vi "GermanInfo_settings_ut_test.vi"(8 "Error In":errorcluster, 11 "Germaninfo in":T1 {"Окно с настройками"."scheme" items=["Complete test scheme 1", "Complete test scheme 2", "Complete test scheme 3"]}) -> (0 "Error Out":errorcluster, 3 "Germaninfo out":T1 {"Окно с настройками"."scheme" items=["Complete test scheme 1", "Complete test scheme 2", "Complete test scheme 3"]})   [LabVIEW 2018]
uses:
  GermanInfo.ctl
  MOKO_LabViewLibrary/MokoSTM/MokoClassicUtilitySTM/MCUS_STM.ctl
  MOKO_LabViewLibrary/MokoSTM/MokoClassicUtilitySTM/MCUS_ITEM.ctl
  <vilib>/addons/_JKI.lib/Serialization/JSON/JKI JSON Serialization.lvlib
panel:
  in  "Iout_EL":dbl=1.0
  in  "Uout_EL":dbl=1.0
  in  "Iin_PS":dbl=1.0
  in  "Reset":bool
  in  "Open":bool
  in  "Save":bool
  in  "Setting Path":path
  in  "Применить":bool
  in  "Uin_PS":dbl=1.0
  in  "Scheme":u16(ring) items=["Complete test scheme 1", "Complete test scheme 2", "Complete test scheme 3"]
  # "Входное напряжение (Uin_PS):"
  # "Входной ток (Iin_PS):"
  # "0,4\n0,6\n1\n1,5\n1,6\n2,5\n4"
  # "kPa\nbar\nkgf/cm2\nMPa"
  # "Выходное напряжение (Uout_EL):"
  # "Выходной ток (Iout_EL):"
  # "Схема измерений:"
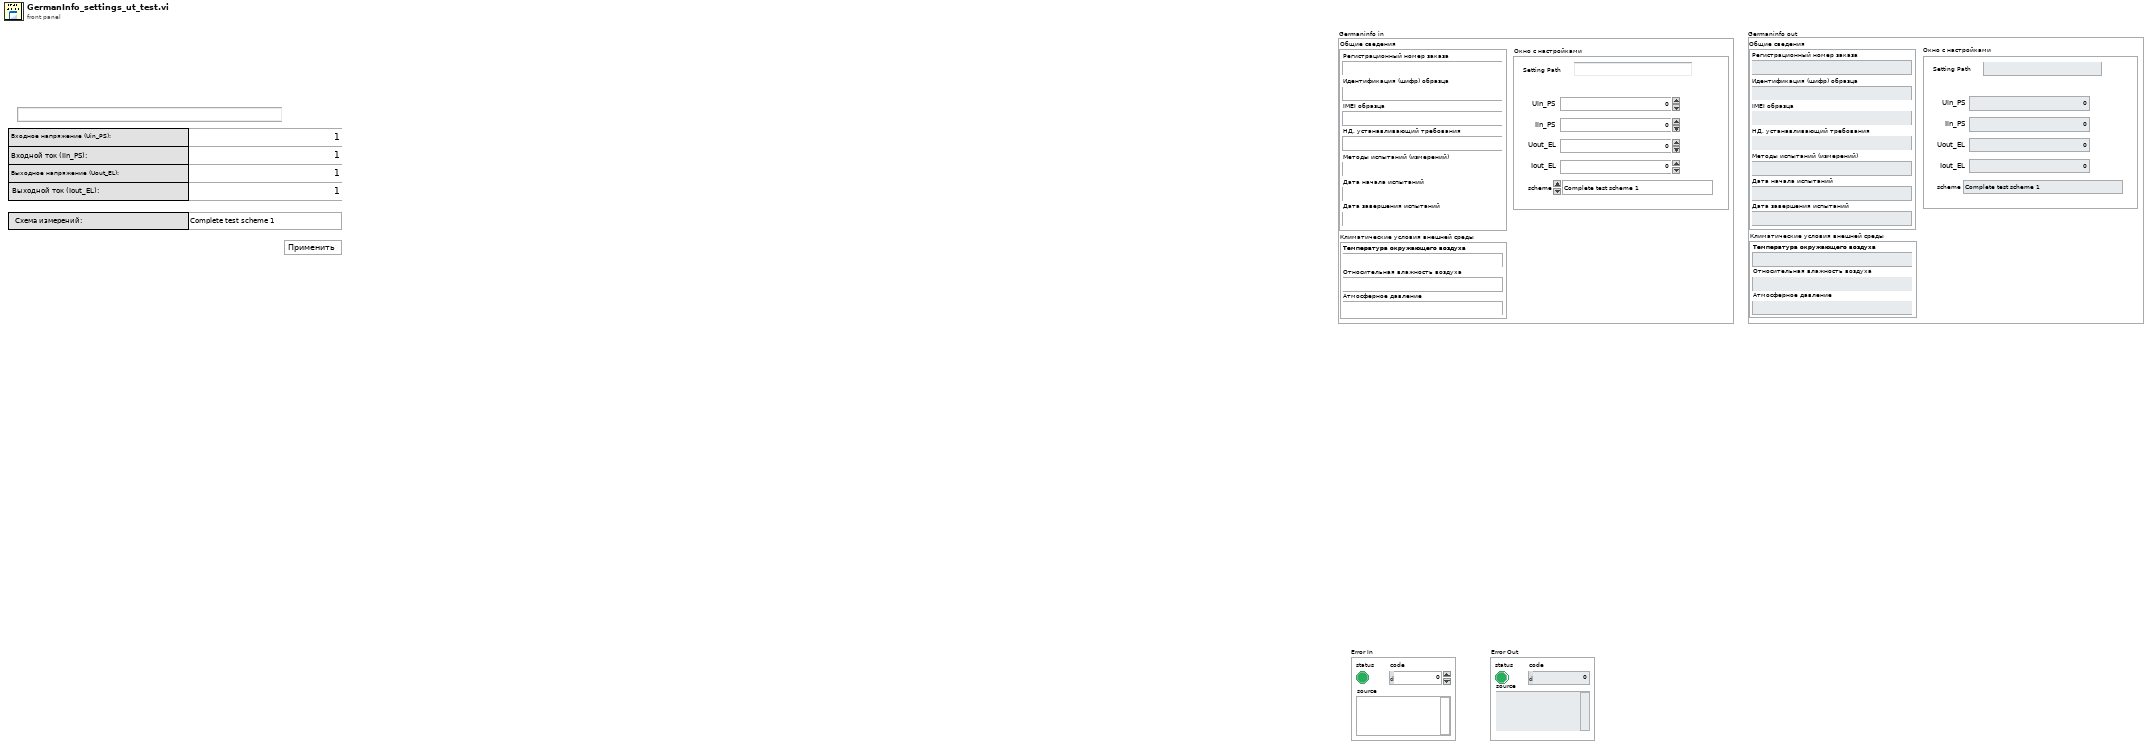
[diagram p1: front panel]
types:
  T1 = typedef "GermanInfo.ctl" = cluster{"Общие сведения":cluster{"Регистрационный номер заказа":string, "Идентификация (шифр) образца":string, "IMEI образца":string, "НД, устанавливающий требования":string, "Методы испытаний (измерений)":string, "Дата начала испытаний":string, "Дата завершения испытаний":string}, "Климатические условия внешней среды":cluster{"Температура окружающего воздуха":string, "Относительная влажность воздуха":string, "Атмосферное давление":string}, "Окно с настройками":cluster{"Uin_PS":dbl, "Setting Path":path, "Iin_PS":dbl, "Uout_EL":dbl, "Iout_EL":dbl, "scheme":u16}}
  T2 = typedef "MCUS_STM.ctl" = cluster{"main stm":T3, "data":string}
  T3 = typedef "MCUS_ITEM.ctl" = enum16{"idle", "_____ main_____ ", "Init", "Stop", "Apply values", "Save", "Open", "Reset"}
  T4 = cluster{"Uin_PS":dbl, "Setting Path":path, "Iin_PS":dbl, "Uout_EL":dbl, "Iout_EL":dbl, "scheme":u16}
  T5 = enum16{"open", "replace", "create", "open or create", "replace or create", "replace or create with confirmation"}
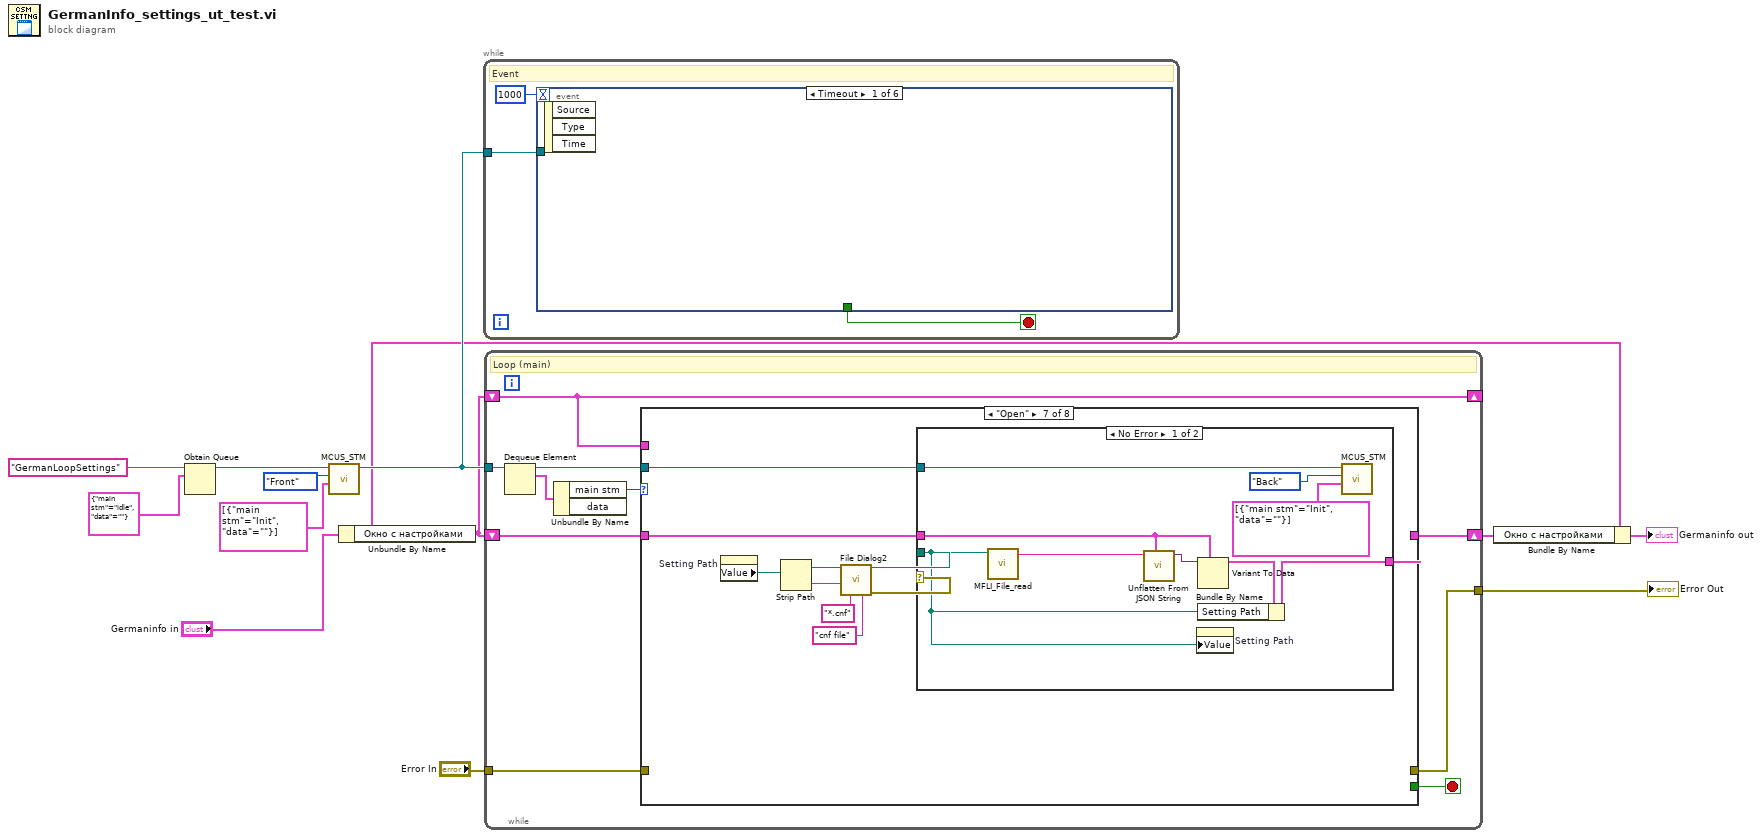
[diagram p0: block diagram]
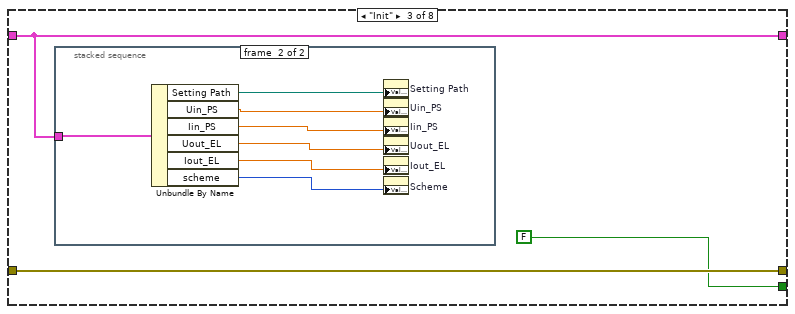
[diagram p4: hidden frame]
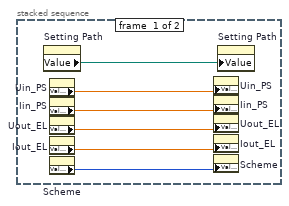
[diagram p5: hidden frame]
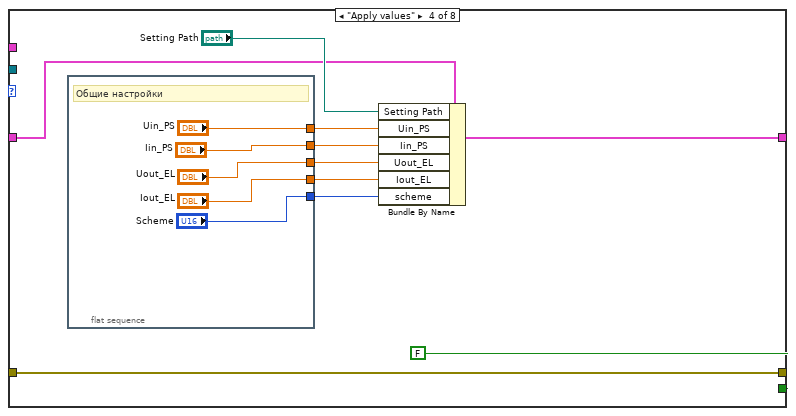
[diagram p6: hidden frame]
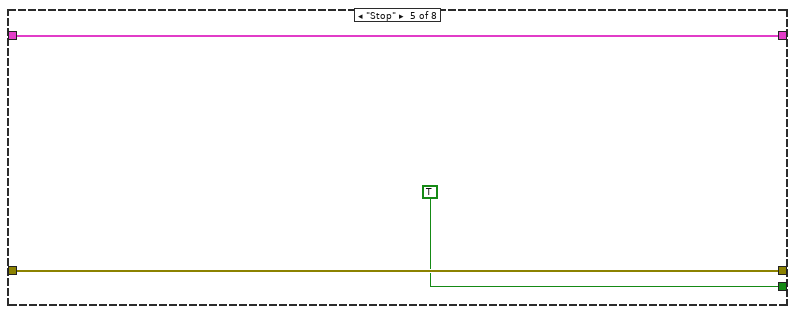
[diagram p7: hidden frame]
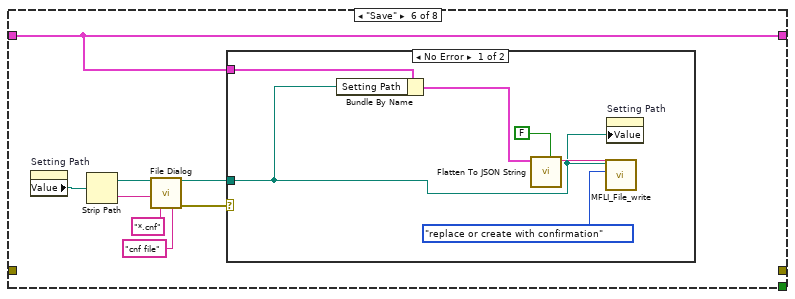
[diagram p8: hidden frame]
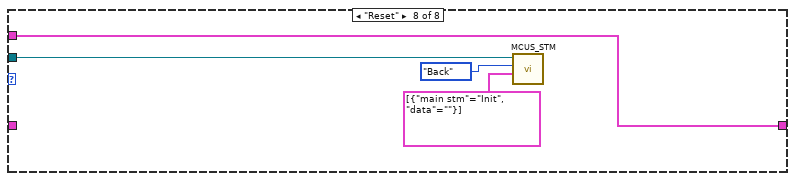
[diagram p11: hidden frame]
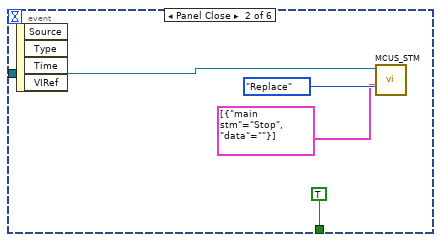
[diagram p12: hidden frame]
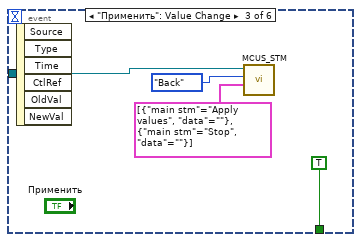
[diagram p13: hidden frame]
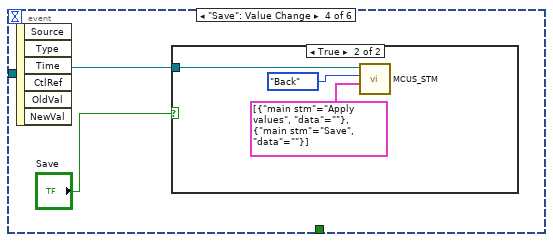
[diagram p14: hidden frame]
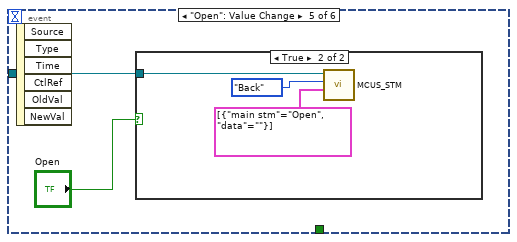
[diagram p16: hidden frame]
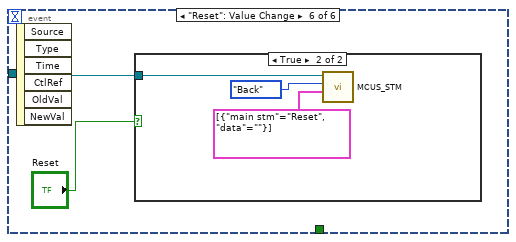
[diagram p18: hidden frame]
diagram:
  n1 = Obtain Queue(name (unnamed)="GermanLoopSettings", element data type=T2 {"main stm"=enum."idle", "data"=""} ("MOKO_NMEA")) -> (queue out=w12:refnum<queue>)  [unwired: 3 in, 2 out]
  n2 = call "MCUS_STM.vi"("StateMachineSteps"=T2[] [{"main stm"=enum."Init", "data"=""}], "FNs"=enum16{"Back", "Front", "Replace"}."Front", "Queue in"=w12) -> ("Queue out"=w7:refnum<queue>)  [unwired: 7 in, 1 out]
  n3 = Unbundle By Name("Germaninfo in") -> ("Окно с настройками"=w4:T4)
  n4 = while {
    tunnel: w7 -> [w13]
    stop <- w15 stop-if-true
    # "Event"
    n5 = event shown="[0] Timeout" {
      selector: _ -> [_ _ _ _ _ _]
      dyn-events: _ -> [_ _ _ _ _ _]
      timeout: 1000 -> [_ _ _ _ _ _]
      tunnel: [_ TRUE TRUE _ _ _] -> w15
      tunnel: w13 -> [_ w16 w21 w25 w30 w35]
      event Timeout {
        n6 = event-data() -> ()  [unwired: 1 in, 3 out]
      }
      event Panel Close {
        n7 = event-data() -> ()  [unwired: 1 in, 4 out]
        n8 = call "MCUS_STM.vi"("StateMachineSteps"=T2[] [{"main stm"=enum."Stop", "data"=""}], "FNs"=enum16{"Back", "Front", "Replace"}."Replace", "Queue in"=w16) -> ()  [unwired: 7 in, 2 out]
      }
      event "Применить": Value Change {
        n9 = event-data() -> ()  [unwired: 1 in, 6 out]
        n10 = call "MCUS_STM.vi"("StateMachineSteps"=T2[] [{"main stm"=enum."Apply values", "data"=""}, {"main stm"=enum."Stop", "data"=""}], "FNs"=enum16{"Back", "Front", "Replace"}."Back", "Queue in"=w21) -> ()  [unwired: 7 in, 2 out]
      }
      event "Save": Value Change {
        n11 = event-data() -> ()  [unwired: 1 in, 6 out]
        n12 = case shown="True" "Save" {
          tunnel: w25 -> [_ w26]
          frame False {
          }
          frame True {
            n13 = call "MCUS_STM.vi"("StateMachineSteps"=T2[] [{"main stm"=enum."Apply values", "data"=""}, {"main stm"=enum."Save", "data"=""}], "FNs"=enum16{"Back", "Front", "Replace"}."Back", "Queue in"=w26) -> ()  [unwired: 7 in, 2 out]
          }
        }
      }
      event "Open": Value Change {
        n14 = event-data() -> ()  [unwired: 1 in, 6 out]
        n15 = case shown="True" "Open" {
          tunnel: w30 -> [_ w31]
          frame False {
          }
          frame True {
            n16 = call "MCUS_STM.vi"("StateMachineSteps"=T2[] [{"main stm"=enum."Open", "data"=""}], "FNs"=enum16{"Back", "Front", "Replace"}."Back", "Queue in"=w31) -> ()  [unwired: 7 in, 2 out]
          }
        }
      }
      event "Reset": Value Change {
        n17 = event-data() -> ()  [unwired: 1 in, 6 out]
        n18 = case shown="True" "Reset" {
          tunnel: w35 -> [_ w36]
          frame False {
          }
          frame True {
            n19 = call "MCUS_STM.vi"("StateMachineSteps"=T2[] [{"main stm"=enum."Reset", "data"=""}], "FNs"=enum16{"Back", "Front", "Replace"}."Back", "Queue in"=w36) -> ()  [unwired: 7 in, 2 out]
          }
        }
      }
    }
  }
  n20 = while {
    tunnel: w7 -> [w48]
    tunnel: "Error In" -> [w44]
    tunnel: [w43] -> w5
    shift-right: [w42] -> w2
    shift-left: w4 -> [w40]
    shift-right: [w39] -> _
    shift-left: w4 -> [w39]
    stop <- w45 stop-if-true
    # "Loop (main)"
    n21 = Dequeue Element(queue=w48) -> (queue out=w41:refnum<queue>, element=w47:T2)  [unwired: 2 in, 2 out]
    n22 = Unbundle By Name(w47) -> ("main stm"=w46:T3)  [unwired: 1 out]
    n23 = case shown="\"Open\"" w46 {
      tunnel: w41 -> [_ _ _ _ _ _ w104 w121]
      tunnel: [_ _ FALSE FALSE TRUE _ _ _] -> w45
      tunnel: w44 -> [w50 w52 w55 w78 w86 _ _ _]
      tunnel: [w50 w52 w55 w78 w86 _ _ _] -> w43
      tunnel: [w49 w51 w53 w76 w84 w90 w106 w124] -> w42
      tunnel: w40 -> [w49 w51 w53 w74 w84 w90 w105 _]
      tunnel: w39 -> [_ _ _ _ _ _ _ w124]
      frame "idle", Default {
      }
      frame "_____ main_____ " {
      }
      frame "Init" {
        n24 = stacked-sequence {
          tunnel: w53 -> [_ w68]
          frame #0 {
            n25 = property on="Setting Path" class="Path"() -> ("Value"=w61:path)  [unwired: 2 in, 2 out]
            n26 = property on="Uin_PS" class="DigNum (strict)"() -> ("Value"=w56:dbl)  [unwired: 2 in, 2 out]
            n27 = property on="Iin_PS" class="DigNum (strict)"() -> ("Value"=w57:dbl)  [unwired: 2 in, 2 out]
            n28 = property on="Uout_EL" class="DigNum (strict)"() -> ("Value"=w58:dbl)  [unwired: 2 in, 2 out]
            n29 = property on="Iout_EL" class="DigNum (strict)"() -> ("Value"=w59:dbl)  [unwired: 2 in, 2 out]
            n30 = property on="Scheme" class="Ring (strict)"() -> ("Value"=w60:u16)  [unwired: 2 in, 2 out]
            n31 = property on="Uin_PS" class="DigNum (strict)"("Value"=w56) -> ()  [unwired: 2 in, 2 out]
            n32 = property on="Iin_PS" class="DigNum (strict)"("Value"=w57) -> ()  [unwired: 2 in, 2 out]
            n33 = property on="Uout_EL" class="DigNum (strict)"("Value"=w58) -> ()  [unwired: 2 in, 2 out]
            n34 = property on="Iout_EL" class="DigNum (strict)"("Value"=w59) -> ()  [unwired: 2 in, 2 out]
            n35 = property on="Scheme" class="Ring (strict)"("Value"=w60) -> ()  [unwired: 2 in, 2 out]
            n36 = property on="Setting Path" class="Path"("Value"=w61) -> ()  [unwired: 2 in, 2 out]
          }
          frame #1 {
            n37 = Unbundle By Name(w68) -> ("Setting Path"=w67:path, "Uin_PS"=w65:dbl, "Iin_PS"=w64:dbl, "Uout_EL"=w63:dbl, "Iout_EL"=w62:dbl, "scheme"=w66:u16)
            n38 = property on="Setting Path" class="Path"("Value"=w67) -> ()  [unwired: 2 in, 2 out]
            n39 = property on="Uin_PS" class="DigNum (strict)"("Value"=w65) -> ()  [unwired: 2 in, 2 out]
            n40 = property on="Iin_PS" class="DigNum (strict)"("Value"=w64) -> ()  [unwired: 2 in, 2 out]
            n41 = property on="Uout_EL" class="DigNum (strict)"("Value"=w63) -> ()  [unwired: 2 in, 2 out]
            n42 = property on="Iout_EL" class="DigNum (strict)"("Value"=w62) -> ()  [unwired: 2 in, 2 out]
            n43 = property on="Scheme" class="Ring (strict)"("Value"=w66) -> ()  [unwired: 2 in, 2 out]
          }
        }
      }
      frame "Apply values" {
        n44 = flat-sequence {
          tunnel: ["Scheme"] -> w73
          tunnel: ["Uin_PS"] -> w72
          tunnel: ["Iin_PS"] -> w71
          tunnel: ["Uout_EL"] -> w70
          tunnel: ["Iout_EL"] -> w69
          frame #0 {
            # "Общие настройки"
          }
        }
        n45 = Bundle By Name(cluster=w74, "Setting Path"="Setting Path", "Uin_PS"=w72, "Iin_PS"=w71, "Uout_EL"=w70, "Iout_EL"=w69, "scheme"=w73) -> (w76:T4)
      }
      frame "Stop" {
      }
      frame "Save" {
        n46 = property on="Setting Path" class="Path"() -> ("Value"=w89:path)  [unwired: 2 in, 2 out]
        n47 = Strip Path(path=w89) -> (stripped path=w88:path, name=w87:string)
        n48 = call "File Dialog"("start path"=w88, "default name"=w87, "pattern (all files)"="*.cnf", "pattern label"="cnf file") -> ("selected path"=w92:path, "error out"=w91:errorcluster)  [unwired: 8 in, 2 out]
        n49 = case shown="No Error" w91 {
          tunnel: w90 -> [w97 _]
          tunnel: w92 -> [w96 _]
          frame No Error {
            n50 = Bundle By Name(cluster=w97, "Setting Path"=w96) -> (w95:T4)
            n51 = call <vilib>:"Flatten To JSON String.vi"("Numeric Extensions (F)"=FALSE, "Variant"=w95) -> ("JSON String"=w99:string)  [unwired: 8 in, 1 out]
            n52 = call "MFLI_File_write.vi"("String"=w99, "operation (0:open)"=T5."replace or create with confirmation", "selected path"=w96) -> ()  [unwired: 7 in, 2 out]
            n53 = property on="Setting Path" class="Path"("Value"=w96) -> ()  [unwired: 2 in, 2 out]
          }
          frame Error {
          }
        }
      }
      frame "Open" {
        n54 = property on="Setting Path" class="Path"() -> ("Value"=w103:path)  [unwired: 2 in, 2 out]
        n55 = Strip Path(path=w103) -> (stripped path=w101:path, name=w102:string)
        n56 = call "File Dialog2"("start path"=w101, "default name"=w102, "pattern (all files)"="*.cnf", "pattern label"="cnf file") -> ("selected path"=w108:path, "error out"=w107:errorcluster)  [unwired: 8 in, 2 out]
        n57 = case shown="No Error" w107 {
          tunnel: w108 -> [w111 _]
          tunnel: w104 -> [w117 _]
          tunnel: w105 -> [w115 w120]
          tunnel: [w112 w120] -> w106
          frame No Error {
            n58 = call "MFLI_File_read.vi"("Project script or program"=w111) -> ("String"=w116:string)  [unwired: 9 in, 1 out]
            n59 = call <vilib>:"Unflatten From JSON String.vi"("Type and Defaults"=w115, "JSON String"=w116) -> ("Variant"=w114:variant)  [unwired: 8 in, 1 out]
            n60 = property on="Setting Path" class="Path"("Value"=w111) -> ()  [unwired: 2 in, 2 out]
            n61 = Variant To Data(type=w115, Variant=w114) -> (data=w113:T4)  [unwired: 1 in, 1 out]
            n62 = Bundle By Name(cluster=w113, "Setting Path"=w111) -> (w112:T4)
            n63 = call "MCUS_STM.vi"("StateMachineSteps"=T2[] [{"main stm"=enum."Init", "data"=""}], "FNs"=enum16{"Back", "Front", "Replace"}."Back", "Queue in"=w117) -> ()  [unwired: 7 in, 2 out]
          }
          frame Error {
          }
        }
      }
      frame "Reset" {
        n64 = call "MCUS_STM.vi"("StateMachineSteps"=T2[] [{"main stm"=enum."Init", "data"=""}], "FNs"=enum16{"Back", "Front", "Replace"}."Back", "Queue in"=w121) -> ()  [unwired: 7 in, 2 out]
      }
    }
  }
  "Error Out" <- w5
  n65 = Bundle By Name(cluster="Germaninfo in", "Окно с настройками"=w2) -> (→"Germaninfo out":T1)
